vi "XML Set Node Text Content.vi"(8 "error in (no error)":errorcluster, 9 "node text":string, 10 "node in":refnum<k20>, 11 "DOM in":refnum<k20>) -> (0 "error out":errorcluster, 2 "node out":refnum<k20>, 3 "DOM out":refnum<k20>)   [LabVIEW 2011, in "COSYLib.lvlib"]
doc: "Returns the combined values of <B>Text_Node</B> children that the <B>node in</B> node owns."
uses:
  <vilib>/xml/Close Reference(Node).vi
  COSYLib.lvlib
  <vilib>/xml/NI_XML.lvlib
  C:/Program Files (x86)/National Instruments/LabVIEW 2011/resource/objmgr/DOMUserDefRef.rc
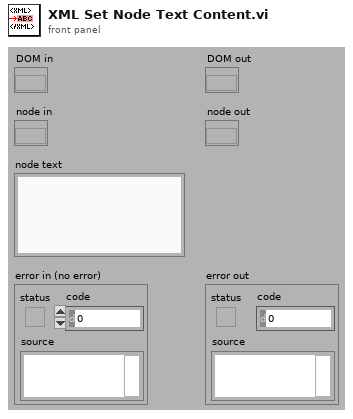
[diagram p1: front panel]
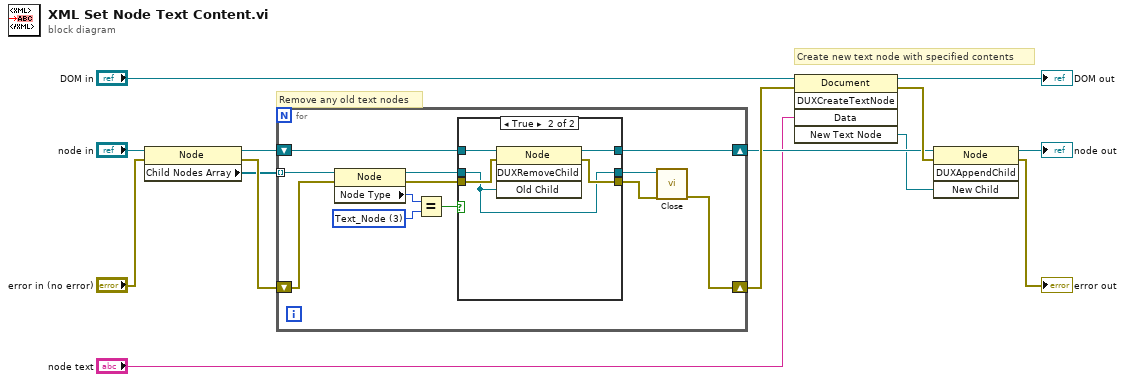
[diagram p0: block diagram]
diagram:
  # "Create new text node with specified contents"
  # "Remove any old text nodes"
  n1 = property class="Node"(reference="node in", error in="error in (no error)") -> (reference out=w7:refnum<k20>, error out=w13:errorcluster, "Child Nodes Array"=w8:refnum<k20>[])
  n2 = for {
    shift-right: [w23] -> w12
    shift-left: w13 -> [w26]
    tunnel: w8 -> [w22] mode=indexing
    shift-right: [w15] -> w6
    shift-left: w7 -> [w16]
    w20 = 3 items=["Element_Node"=1, "Attribute_Node"=2, "Text_Node"=3, "CDATASection_Node"=4, "EntityReference_Node"=5, "Entity_Node"=6, "ProcessingInstruction_Node"=7, "Comment_Node"=8, "Document_Node"=9, "DocumentType_Node"=10, "DocumentFragment_Node"=11, "Notation_Node"=12] ("Node Type")
    n3 = property class="Node"(reference=w22, error in=w26) -> (reference out=w18:refnum<k20>, error out=w25:errorcluster, "Node Type"=w21:i32)
    n4 = Equal?(x=w21, y=w20) -> (x = y?=w19:bool)
    n5 = case shown="True" w19 {
      tunnel: w18 -> [w28 w31]
      tunnel: w25 -> [w29 w34]
      tunnel: [w28 w31] -> w17
      tunnel: [w29 w33] -> w24
      tunnel: w16 -> [w27 w32]
      tunnel: [w27 w30] -> w15
      frame False {
      }
      frame True {
        n6 = invoke class="Node" method="DUXRemoveChild"(reference=w32, error in=w34, "Old Child"=w31) -> (reference out=w30:refnum<k20>, error out=w33:errorcluster)  [unwired: 1 in, 2 out]
      }
    }
    n7 = call-poly <vilib>:"Close.vi"("error in (no error)"=w24, "node"=w17) -> ("error out"=w23:errorcluster)  [unwired: 7 out]
  }
  n8 = invoke class="Document" method="DUXCreateTextNode"(reference="DOM in", error in=w12, "Data"="node text") -> (reference out=→"DOM out":refnum<k20>, error out=w11:errorcluster, "New Text Node"=w2:refnum<k20>)  [unwired: 2 in, 2 out]
  n9 = invoke class="Node" method="DUXAppendChild"(reference=w6, error in=w11, "New Child"=w2) -> (reference out=→"node out":refnum<k20>, error out=→"error out":errorcluster)  [unwired: 1 in, 2 out]
